vi "Delta Time.vi"(11 "Element in":refnum<class "Element.lvclass">) -> (2 "Last Time":dbl format="%.3f")   [LabVIEW 2021, in "Element.lvclass"]
uses:
  Element.lvclass
  Element.lvclass/Element.ctl
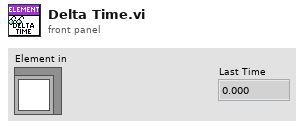
[diagram p1: front panel]
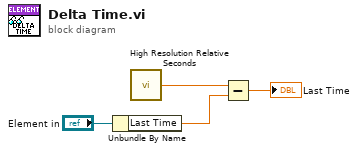
[diagram p0: block diagram]
diagram:
  n1 = Unbundle By Name("Element in") -> ("Last Time"=w2:dbl)
  n2 = call <vilib>:"High Resolution Relative Seconds.vi"() -> ("relative seconds"=w3:dbl)
  n3 = Subtract(x=w3, y=w2) -> (x-y=→"Last Time":dbl)
